vi "Set-Image-offset-x.vi"(8 "error in (no error)":errorcluster, 9 "Offset X in":i32, 10 "Image width":i32, 11 "PF_MV1-D1312-240 in":refnum<class "PF_MV1-D1312-240.lvclass">) -> (0 "error out":errorcluster, 1 "Offset X":i32, 3 "PF_MV1-D1312-240 out":refnum<class "PF_MV1-D1312-240.lvclass">)   [LabVIEW 2013, in "CameraVision.lvlib" / "PF_MV1-D1312-240.lvclass"]
uses:
  PF_MV1-D1312-240.lvclass
  Camera.lvclass/Camera.ctl
  Read IMAQ Session.vi
  <userlib>/Photonfocus Toolkit/_Public/SubVIs/pf_Set_Camera_Property_Int.vi
  <userlib>/Photonfocus Toolkit/Photonfocus_Toolkit.lvlib
  Camera.lvclass
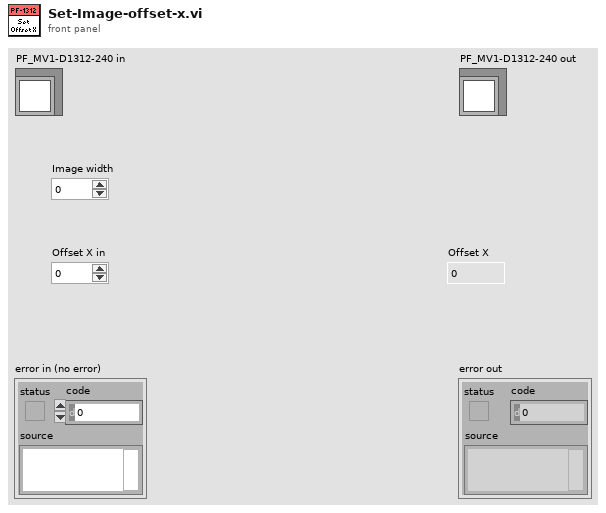
[diagram p1: front panel]
types:
  T1 = cluster{"Max. offset X":i32, "Max. offset Y":i32, "Offset step size X":i32, "Offset step size Y":i32}
  T2 = cluster{"Max. width":i32, "Max. height":i32, "Step size width":dbl, "Min. width":i32, "Min. height":i32, "Step size height":dbl}
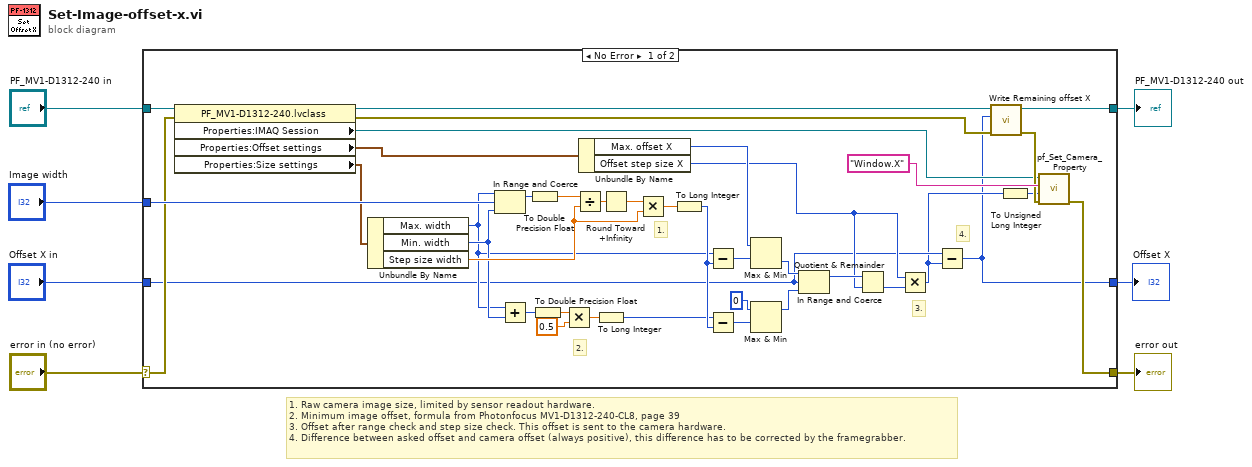
[diagram p0: block diagram]
diagram:
  # "1. Raw camera image size, limited by sensor readout hardware.\n2. Minimum image offset, formula from Photonfocus MV1-D1312-240-CL8, page 39\n3. Offset after range check and step size check. This offset is sent to the camera hardware.\n4. Difference between asked offset and camera offset (always positive), this difference has to be corrected by the framegrabber."
  n1 = case shown="No Error" "error in (no error)" {
    selector: "error in (no error)" -> [w29 w49]
    tunnel: [w45 w49] -> w6
    tunnel: [w14 w48] -> w4
    tunnel: "PF_MV1-D1312-240 in" -> [w46 w48]
    tunnel: "Image width" -> [w43 _]
    tunnel: [w9 w47] -> w2
    tunnel: "Offset X in" -> [w17 w47]
    frame No Error {
      # "4."
      # "3."
      # "2."
      # "1."
      n2 = property class="PF_MV1-D1312-240.lvclass"(reference=w46, error in=w29) -> (reference out=w15:refnum<class "PF_MV1-D1312-240.lvclass">, error out=w12:errorcluster, "Properties:IMAQ Session"=w11:refnum<k11>, "Properties:Offset settings"=w16:T1, "Properties:Size settings"=w28:T2)
      n3 = Unbundle By Name(w28) -> ("Max. width"=w25:i32, "Min. width"=w26:i32, "Step size width"=w27:dbl)
      n4 = In Range and Coerce(upper limit=w25, x=w43, lower limit=w26) -> (coerced(x)=w31:i32)  [unwired: 1 out]
      n5 = Add(x=w25, y=w26) -> (x+y=w24:i32)
      n6 = To Double Precision Float(number=w31) -> (double precision float=w32:dbl)
      n7 = To Double Precision Float(number=w24) -> (double precision float=w22:dbl)
      n8 = Multiply(x=w22, y=0.5) -> (x*y=w21:dbl)
      n9 = Divide(x=w32, y=w27) -> (x/y=w34:dbl)
      n10 = Unbundle By Name(w16) -> ("Max. offset X"=w19:i32, "Offset step size X"=w18:i32)
      n11 = To Long Integer(number=w21) -> (32bit integer=w20:i32)
      n12 = Round Toward +Infinity(x=w34) -> (ceil(x): smallest int >= x=w33:dbl)
      n13 = Multiply(x=w33, y=w27) -> (x*y=w35:dbl)
      n14 = To Long Integer(number=w35) -> (32bit integer=w30:i32)
      n15 = Subtract(x=w25, y=w30) -> (x-y=w42:i32)
      n16 = Subtract(x=w20, y=w30) -> (x-y=w40:i32)
      n17 = Max & Min(x=w19, y=w42) -> (min(x,y)=w41:i32)  [unwired: 1 out]
      n18 = Max & Min(x=0, y=w40) -> (max(x,y)=w38:i32)  [unwired: 1 out]
      n19 = In Range and Coerce(upper limit=w41, x=w17, lower limit=w38) -> (coerced(x)=w36:i32)  [unwired: 1 out]
      n20 = Quotient & Remainder(x=w36, y=w18) -> (floor(x/y)=w37:i32)  [unwired: 1 out]
      n21 = Multiply(x=w18, y=w37) -> (x*y=w10:i32)
      n22 = Subtract(x=w17, y=w10) -> (x-y=w9:i32)
      n23 = call "Write Remaining offset X.vi"("error in (no error)"=w12, "Offset X"=w9, "Camera in"=w15) -> ("error out"=w13:errorcluster, "Camera out"=w14:refnum<class "PF_MV1-D1312-240.lvclass">)  [unwired: 7 in]
      n24 = To Unsigned Long Integer(number=w10) -> (unsigned 32bit integer=w8:u32)
      n25 = call-poly <userlib>:"pf_Set_Camera_Property.vi"("error in (no error)"=w13, "Property Value"=w8, "Property Name"="Window.X", "IMAQ Session in"=w11) -> ("error out"=w45:errorcluster)  [unwired: 5 in, 2 out]
    }
    frame Error {
    }
  }
  "error out" <- w6
  "PF_MV1-D1312-240 out" <- w4
  "Offset X" <- w2
